vi "ExtractArchivedData.vi"() -> ()   [LabVIEW 2013, in "examples.lvlib"]
uses:
  examples.lvlib
  vis/lv-2013/tango_vi.llb/avToDoubleScalarAv.vi
  vis/lv-2013/tango_vi.llb/tango.lvlib
panel:
  out "success":bool
  out "XY Graph":cluster{"Y":dbl[], "Y":dbl[]}[](graph)
  in  "sampling":string="MINUTE"
  in  "to_date":string="2010-02-02 00:00:00"
  in  "from_date":string="2010-02-01 00:00:00"
  in  "archived_attr_name":string="ANS-C03/DG/DCCT/current"
  in  "db_extractor_dev_name":string="archiving/hdbextractor/1"
  out "archived values":dbl[][](array[numeric])
  out "timestamps":dbl[][](array[numeric])
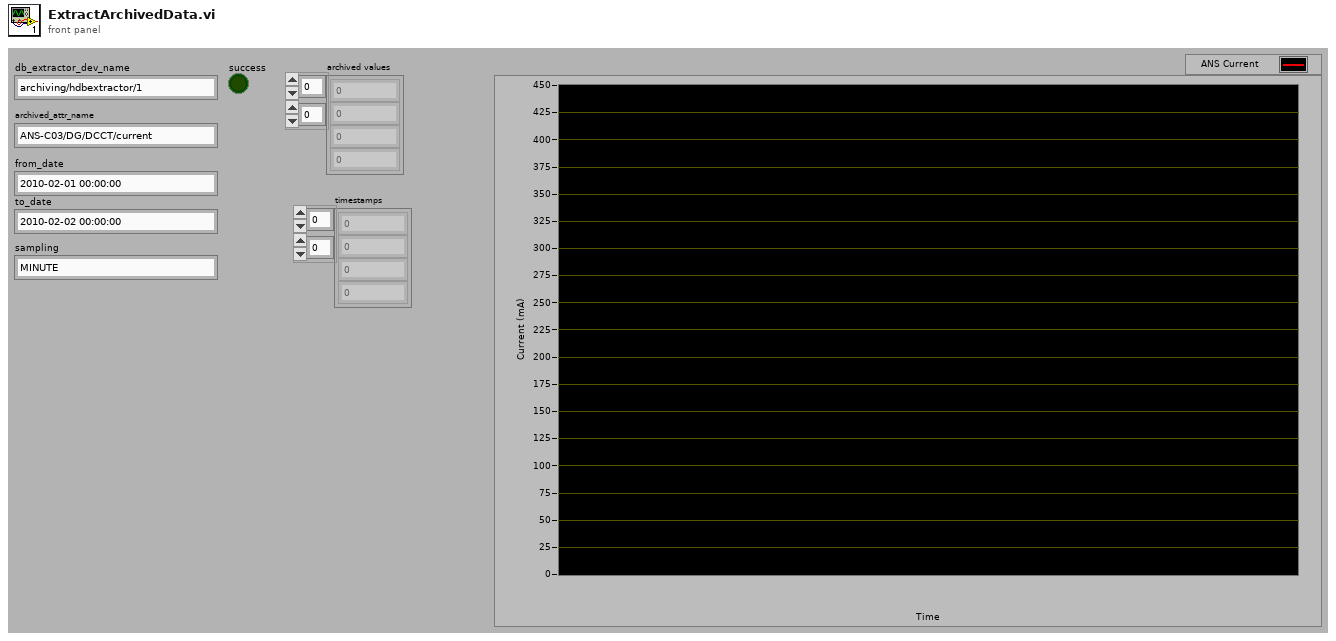
[diagram p1: front panel]
types:
  T1 = cluster{"device name":string, "attribute name":string, "quality value":i16, "quality string":string, "timestamp":dbl, "dim. x":i32, "dim. y":i32, "value":u8[], "error code":i32, "error stack":string[], "data type":u16}[]
  T2 = cluster{"device name":string, "attribute name":string, "quality value":i16, "quality string":string, "timestamp":dbl, "dim. x":i32, "dim. y":i32, "value":dbl, "error code":i32, "error stack":string[], "data type":u16}
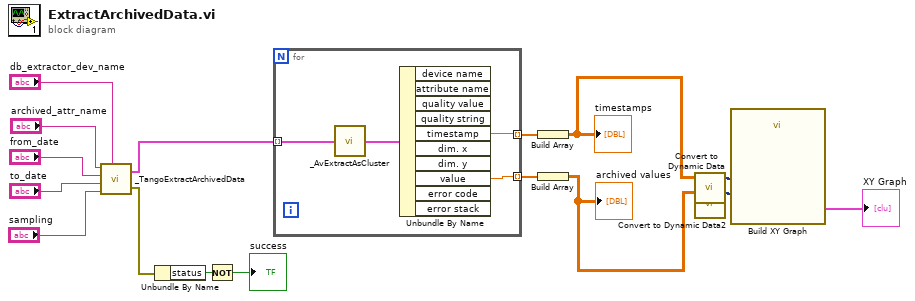
[diagram p0: block diagram]
diagram:
  n1 = call "_TangoExtractArchivedData.vi"("db_extractor_dev_name"="db_extractor_dev_name", "sampling"="sampling", "to_date"="to_date", "from_date"="from_date", "archived_attr_name"="archived_attr_name") -> ("error out"=w3:errorcluster, "attr values"=w11:T1)  [unwired: 1 in]
  n2 = Unbundle By Name(w3) -> ("status"=w2:bool)
  n3 = Not(x=w2) -> (.not. x?=→"success":bool)
  n4 = for {
    tunnel: w11 -> [w20] mode=indexing
    tunnel: [w18] -> w7 mode=indexing
    tunnel: [w17] -> w5 mode=indexing
    n5 = call-poly "_AvExtractAsCluster.vi"("attribute value"=w20) -> ("av"=w19:T2)
    n6 = Unbundle By Name(w19) -> ("timestamp"=w18:dbl, "value"=w17:dbl)  [unwired: 8 out]
  }
  n7 = Build Array(w7) -> (w6:dbl[][])
  "timestamps" <- w6
  n8 = Build Array(w5) -> (w4:dbl[][])
  "archived values" <- w4
  n9 = call "Convert to Dynamic Data"("2D Array"=w6) -> ("Dynamic Data Type"=w9:dynamicdata)  [unwired: 3 in]
  n10 = call "Convert to Dynamic Data2"("2D Array"=w4) -> ("Dynamic Data Type"=w8:dynamicdata)  [unwired: 3 in]
  n11 = call "Build XY Graph"("Y Input"=w8, "X Input"=w9) -> ("XY Graph"=→"XY Graph":cluster{"Y":dbl[], "Y":dbl[]}[])  [unwired: 8 in, 1 out]
